vi "Prepare Acquisition.vi"(8 "error in (no error)":errorcluster, 10 "Flash Settings":T1={"Exposure Time (ms)"=100.0, "Binning"=enum."2x2", "Scan Mode"=0, "Frames to Acquire"=1000.0, "Pixel Correction"=FALSE, "Frames to Skip"=0, "File Path"=path "", "Duty cycle"=0.0, "ALEX"=FALSE, "Shutter Enable"=[], "fluidics trigger frame"=0, "Bit Depth"=0, "Image Width (px)"=0, "Image Height (px)"=0, "Horizontal Offset (px)"=0, "Vertical Offset (px)"=0} {"fluidics trigger frame" max=60000 step=1; "Exposure Time (ms)" min=1.0 max=10000.0 step=1.0}, 11 "Orca-Flash 4.0 in":refnum<class "Hamamatsu Camera.lvclass">) -> (0 "error out":errorcluster, 3 "Orca-Flash 4.0 out":refnum<class "Hamamatsu Camera.lvclass">)   [LabVIEW 2023, in "Hamamatsu Camera.lvlib" / "Hamamatsu Camera.lvclass"]
uses:
  Hamamatsu Camera.lvclass
  Resources/Type Defs/Camera Settings.ctl
  Hamamatsu Camera.lvclass/Hamamatsu Camera.ctl
  Resources/GLOBAL/GLOBAL Experiment Metadata.vi
  Resources/GLOBAL/GLOBAL Debug.vi
  Resources/GLOBAL/GLOBAL Time-critical.vi
  Hamamatsu Camera.lvlib
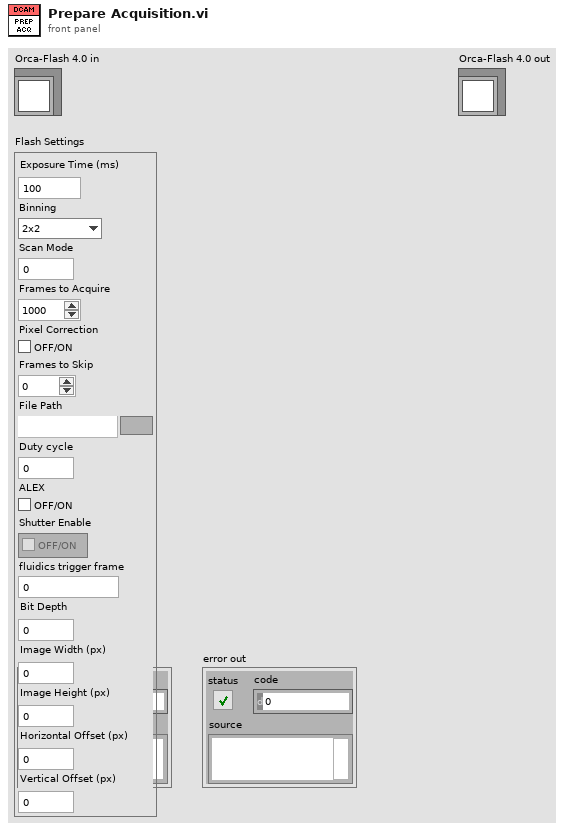
[diagram p1: front panel]
types:
  T1 = typedef "Camera Settings.ctl" = cluster{"Exposure Time (ms)":dbl, "Binning":enum16{"1x1", "2x2", "4x4"}, "Scan Mode":i32, "Frames to Acquire":dbl, "Pixel Correction":bool, "Frames to Skip":u32, "File Path":path, "Duty cycle":dbl, "ALEX":bool, "Shutter Enable":bool[], "fluidics trigger frame":u16, "Bit Depth":u16, "Image Width (px)":u16, "Image Height (px)":u16, "Horizontal Offset (px)":u16, "Vertical Offset (px)":u16}
  T2 = cluster{"Horizontal Offset":i32, "Vertical Offset":i32, "Horizontal Size":i32, "Vertical Size":i32}
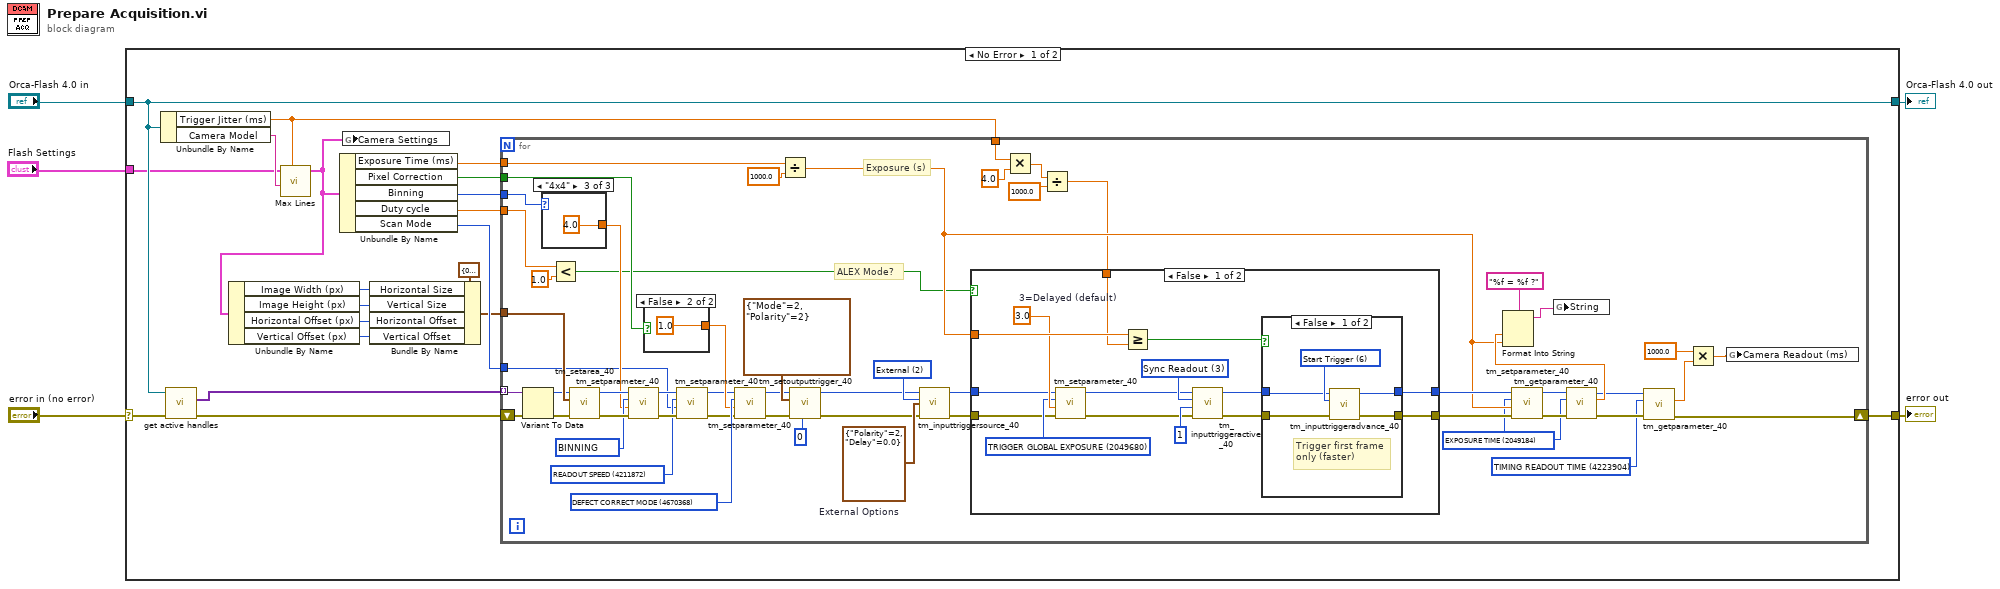
[diagram p0: block diagram]
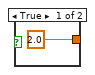
[diagram p2: hidden frame]
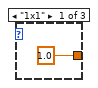
[diagram p3: hidden frame]
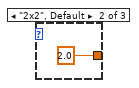
[diagram p4: hidden frame]
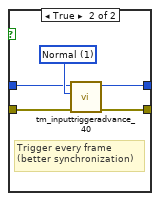
[diagram p5: hidden frame]
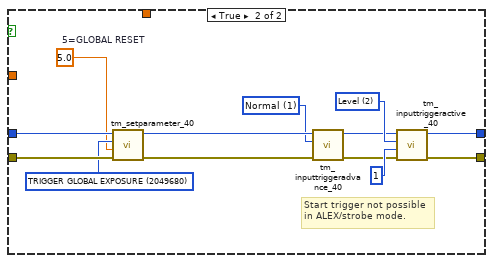
[diagram p6: hidden frame]
diagram:
  n1 = case shown="No Error" "error in (no error)" {
    selector: "error in (no error)" -> [w20 w125]
    tunnel: [w25 w125] -> w3
    tunnel: "Flash Settings" -> [w14 _]
    tunnel: "Orca-Flash 4.0 in" -> [w16 w124]
    tunnel: [w16 w124] -> w1
    frame No Error {
      n2 = Unbundle By Name(w16) -> ("Trigger Jitter (ms)"=w6:dbl, "Camera Model"=w15:string)
      n3 = call-dynamic "get active handles.vi"("error in (no error)"=w20, "Camera in"=w16) -> ("error out"=w21:errorcluster, "Handles"=w22:variant[])  [unwired: 5 in, 3 out]
      n4 = call "Max Lines.vi"("Trigger Jitter (ms)"=w6, "Camera Model"=w15, "Camera Setings In"=w14) -> ("Camera Settings Out"=w11:T1)  [unwired: 7 in, 1 out]
      n5 = Unbundle By Name(w11) -> ("Image Width (px)"=w10:u16, "Image Height (px)"=w9:u16, "Horizontal Offset (px)"=w8:u16, "Vertical Offset (px)"=w7:u16)
      n6 = Unbundle By Name(w11) -> ("Exposure Time (ms)"=w17:dbl, "Pixel Correction"=w24:bool, "Binning"=w23:enum16{"1x1", "2x2", "4x4"}, "Duty cycle"=w18:dbl, "Scan Mode"=w13:i32)
      n7 = global write "GLOBAL Experiment Metadata.vi" "Camera Settings"(w11) -> ()
      n8 = Bundle By Name(cluster=T2 {"Horizontal Offset"=0, "Vertical Offset"=0, "Horizontal Size"=0, "Vertical Size"=0} ("Sub Region"), "Horizontal Size"=w10, "Vertical Size"=w9, "Horizontal Offset"=w8, "Vertical Offset"=w7) -> (w12:T2)
      n9 = for {
        shift-right: [w34] -> w25
        shift-left: w21 -> [w41]
        tunnel: w22 -> [w39] mode=indexing
        tunnel: w17 -> [w49]
        tunnel: w24 -> [w48]
        tunnel: w23 -> [w47]
        tunnel: w18 -> [w46]
        tunnel: w12 -> [w43]
        tunnel: w13 -> [w42]
        tunnel: w6 -> [w28]
        w35 = u32 4223904 items=["SENSOR MODE"=4212128, "SENSOR MODE LINE BUNDLE HEIGHT"=4212192, "READOUT DIRECTION"=4211904, "BIT PER CHANNEL"=4342976, "EXPOSURE TIME"=2049184, "CONTRAST GAIN"=3163312, "BINNING"=4215968, "TIMING READOUT TIME"=4223904, "INTERNAL FRAME RATE"=4225952, "INTERNAL FRAME INTERVAL"=4225968, "INTERNAL LINE SPEED"=4226000, "IMAGE WIDTH"=4343200, "IMAGE HEIGHT"=4343216, "IMAGE ROWBYTES"=4343232, "IMAGE FRAMEBYTES"=4343248, "IMAGE PIXEL TYPE"=4343296] ("Parameter")
        w44 = u32 2049184 items=["SENSOR MODE"=4212128, "READOUT SPEED"=4211872, "READOUT DIRECTION"=4211904, "BIT PER CHANNEL"=4342976, "TRIGGER GLOBAL EXPOSURE"=2049680, "TRIGGER DELAY"=1066480, "SYNC READOUT SYSTEM BLANK"=1066528, "SENSOR COOLER STATUS"=2115280, "EXPOSURE TIME"=2049184, "DEFECT CORRECT MODE"=4670368, "BINNING"=4215968, "TIMING READOUT TIME"=4223904, "INTERNAL FRAME RATE"=4225952, "INTERNAL FRAME INTERVAL"=4225968, "INTERNAL LINE SPEED"=4226000, "INTERNAL LINE INTERVAL"=4226016, "IMAGE WIDTH"=4343200, "IMAGE HEIGHT"=4343216, "IMAGE ROWBYTES"=4343232, "IMAGE FRAMEBYTES"=4343248, "IMAGE PIXEL TYPE"=4343296, "NUMBER OF OUTPUT TRIGGER CONNECTOR"=1852320, "OUTPUT TRIGGER SOURCE[0]"=1852576, "OUTPUT TRIGGER SOURCE[1]"=1852832, "OUTPUT TRIGGER SOURCE[2]"=1853088, "OUTPUT TRIGGER POLARITY[0]"=1852592, "OUTPUT TRIGGER POLARITY[1]"=1852848, "OUTPUT TRIGGER POLARITY[2]"=1853104, "OUTPUT TRIGGER ACTIVE[0]"=1852608, "OUTPUT TRIGGER ACTIVE[1]"=1852864, "OUTPUT TRIGGER ACTIVE[2]"=1853120, "OUTPUT TRIGGER DELAY[0]"=1852624, "OUTPUT TRIGGER DELAY[1]"=1852880, "OUTPUT TRIGGER DELAY[2]"=1853136, "OUTPUT TRIGGER PERIOD[0]"=1852640, "OUTPUT TRIGGER PERIOD[1]"=1852896, "OUTPUT TRIGGER PERIOD[2]"=1853152, "OUTPUT TRIGGER KIND[0]"=1852656, "OUTPUT TRIGGER KIND[1]"=1852912, "OUTPUT TRIGGER KIND[2]"=1853168, "OUTPUT TRIGGER PRE HSYNC COUNT"=1852704] ("Parameter")
        w68 = 2 items=["Internal"=1, "External"=2, "Software"=3, "Master Pulse"=4] ("Source")
        w69 = cluster{"Polarity":i32, "Delay":dbl} {"Polarity"=2, "Delay"=0.0}  # External Options
        w72 = u32 4670368 items=["SENSOR MODE"=4212128, "READOUT SPEED"=4211872, "READOUT DIRECTION"=4211904, "BIT PER CHANNEL"=4342976, "TRIGGER GLOBAL EXPOSURE"=2049680, "TRIGGER DELAY"=1066480, "SYNC READOUT SYSTEM BLANK"=1066528, "SENSOR COOLER STATUS"=2115280, "EXPOSURE TIME"=2049184, "DEFECT CORRECT MODE"=4670368, "BINNING"=4215968, "TIMING READOUT TIME"=4223904, "INTERNAL FRAME RATE"=4225952, "INTERNAL FRAME INTERVAL"=4225968, "INTERNAL LINE SPEED"=4226000, "INTERNAL LINE INTERVAL"=4226016, "IMAGE WIDTH"=4343200, "IMAGE HEIGHT"=4343216, "IMAGE ROWBYTES"=4343232, "IMAGE FRAMEBYTES"=4343248, "IMAGE PIXEL TYPE"=4343296, "NUMBER OF OUTPUT TRIGGER CONNECTOR"=1852320, "OUTPUT TRIGGER SOURCE[0]"=1852576, "OUTPUT TRIGGER SOURCE[1]"=1852832, "OUTPUT TRIGGER SOURCE[2]"=1853088, "OUTPUT TRIGGER POLARITY[0]"=1852592, "OUTPUT TRIGGER POLARITY[1]"=1852848, "OUTPUT TRIGGER POLARITY[2]"=1853104, "OUTPUT TRIGGER ACTIVE[0]"=1852608, "OUTPUT TRIGGER ACTIVE[1]"=1852864, "OUTPUT TRIGGER ACTIVE[2]"=1853120, "OUTPUT TRIGGER DELAY[0]"=1852624, "OUTPUT TRIGGER DELAY[1]"=1852880, "OUTPUT TRIGGER DELAY[2]"=1853136, "OUTPUT TRIGGER PERIOD[0]"=1852640, "OUTPUT TRIGGER PERIOD[1]"=1852896, "OUTPUT TRIGGER PERIOD[2]"=1853152, "OUTPUT TRIGGER KIND[0]"=1852656, "OUTPUT TRIGGER KIND[1]"=1852912, "OUTPUT TRIGGER KIND[2]"=1853168, "OUTPUT TRIGGER PRE HSYNC COUNT"=1852704] ("Parameter")
        w73 = u32 4211872 items=["SENSOR MODE"=4212128, "READOUT SPEED"=4211872, "READOUT DIRECTION"=4211904, "BIT PER CHANNEL"=4342976, "TRIGGER GLOBAL EXPOSURE"=2049680, "TRIGGER DELAY"=1066480, "SYNC READOUT SYSTEM BLANK"=1066528, "SENSOR COOLER STATUS"=2115280, "EXPOSURE TIME"=2049184, "DEFECT CORRECT MODE"=4670368, "BINNING"=4215968, "TIMING READOUT TIME"=4223904, "INTERNAL FRAME RATE"=4225952, "INTERNAL FRAME INTERVAL"=4225968, "INTERNAL LINE SPEED"=4226000, "INTERNAL LINE INTERVAL"=4226016, "IMAGE WIDTH"=4343200, "IMAGE HEIGHT"=4343216, "IMAGE ROWBYTES"=4343232, "IMAGE FRAMEBYTES"=4343248, "IMAGE PIXEL TYPE"=4343296, "NUMBER OF OUTPUT TRIGGER CONNECTOR"=1852320, "OUTPUT TRIGGER SOURCE[0]"=1852576, "OUTPUT TRIGGER SOURCE[1]"=1852832, "OUTPUT TRIGGER SOURCE[2]"=1853088, "OUTPUT TRIGGER POLARITY[0]"=1852592, "OUTPUT TRIGGER POLARITY[1]"=1852848, "OUTPUT TRIGGER POLARITY[2]"=1853104, "OUTPUT TRIGGER ACTIVE[0]"=1852608, "OUTPUT TRIGGER ACTIVE[1]"=1852864, "OUTPUT TRIGGER ACTIVE[2]"=1853120, "OUTPUT TRIGGER DELAY[0]"=1852624, "OUTPUT TRIGGER DELAY[1]"=1852880, "OUTPUT TRIGGER DELAY[2]"=1853136, "OUTPUT TRIGGER PERIOD[0]"=1852640, "OUTPUT TRIGGER PERIOD[1]"=1852896, "OUTPUT TRIGGER PERIOD[2]"=1853152, "OUTPUT TRIGGER KIND[0]"=1852656, "OUTPUT TRIGGER KIND[1]"=1852912, "OUTPUT TRIGGER KIND[2]"=1853168, "OUTPUT TRIGGER PRE HSYNC COUNT"=1852704] ("Parameter")
        w77 = u32 4215968 items=["SENSOR MODE"=4212128, "READOUT SPEED"=4211872, "READOUT DIRECTION"=4211904, "BIT PER CHANNEL"=4342976, "TRIGGER GLOBAL EXPOSURE"=2049680, "TRIGGER DELAY"=1066480, "SYNC READOUT SYSTEM BLANK"=1066528, "SENSOR COOLER STATUS"=2115280, "EXPOSURE TIME"=2049184, "DEFECT CORRECT MODE"=4670368, "BINNING"=4215968, "TIMING READOUT TIME"=4223904, "INTERNAL FRAME RATE"=4225952, "INTERNAL FRAME INTERVAL"=4225968, "INTERNAL LINE SPEED"=4226000, "INTERNAL LINE INTERVAL"=4226016, "IMAGE WIDTH"=4343200, "IMAGE HEIGHT"=4343216, "IMAGE ROWBYTES"=4343232, "IMAGE FRAMEBYTES"=4343248, "IMAGE PIXEL TYPE"=4343296, "NUMBER OF OUTPUT TRIGGER CONNECTOR"=1852320, "OUTPUT TRIGGER SOURCE[0]"=1852576, "OUTPUT TRIGGER SOURCE[1]"=1852832, "OUTPUT TRIGGER SOURCE[2]"=1853088, "OUTPUT TRIGGER POLARITY[0]"=1852592, "OUTPUT TRIGGER POLARITY[1]"=1852848, "OUTPUT TRIGGER POLARITY[2]"=1853104, "OUTPUT TRIGGER ACTIVE[0]"=1852608, "OUTPUT TRIGGER ACTIVE[1]"=1852864, "OUTPUT TRIGGER ACTIVE[2]"=1853120, "OUTPUT TRIGGER DELAY[0]"=1852624, "OUTPUT TRIGGER DELAY[1]"=1852880, "OUTPUT TRIGGER DELAY[2]"=1853136, "OUTPUT TRIGGER PERIOD[0]"=1852640, "OUTPUT TRIGGER PERIOD[1]"=1852896, "OUTPUT TRIGGER PERIOD[2]"=1853152, "OUTPUT TRIGGER KIND[0]"=1852656, "OUTPUT TRIGGER KIND[1]"=1852912, "OUTPUT TRIGGER KIND[2]"=1853168, "OUTPUT TRIGGER PRE HSYNC COUNT"=1852704] ("Parameter")
        # "Exposure (s)"
        # "ALEX Mode?"
        n10 = Variant To Data(error in=w41, Variant=w39) -> (data=w38:u32, error out=w40:errorcluster)  [unwired: 1 in]
        n11 = case shown="\"4x4\"" w47 {
          tunnel: [1.0 ("Value in") 2.0 ("Value in") 4.0 ("Value in")] -> w76
          frame "1x1" {
          }
          frame "2x2", Default {
          }
          frame "4x4" {
          }
        }
        n12 = Less?(x=w46, y=1.0) -> (x < y?=w45:bool)
        n13 = call <userlib>:"tm_setarea_40.vi"("error in (no error)"=w40, "Sub Region"=w43, "Handle in"=w38) -> ("error out"=w79:errorcluster, "Handle out"=w78:u32)  [unwired: 7 in]
        n14 = call <userlib>:"tm_setparameter_40.vi"("error in (no error)"=w79, "Value in"=w76, "Parameter"=w77, "Handle in"=w78) -> ("error out"=w74:errorcluster, "Handle out"=w75:u32)  [unwired: 6 in]
        n15 = case shown="False" w48 {
          tunnel: [sgl 2.0 ("1 = OFF\n2 = ON") sgl 1.0 ("1 = OFF\n2 = ON")] -> w71
          frame True {
          }
          frame False {
          }
        }
        n16 = call <userlib>:"tm_setparameter_40.vi"("error in (no error)"=w74, "Value in"=w42, "Parameter"=w73, "Handle in"=w75) -> ("error out"=w55:errorcluster, "Handle out"=w56:u32)  [unwired: 6 in]
        n17 = call <userlib>:"tm_setparameter_40.vi"("error in (no error)"=w55, "Value in"=w71, "Parameter"=w72, "Handle in"=w56) -> ("error out"=w62:errorcluster, "Handle out"=w63:u32)  [unwired: 6 in]
        n18 = Divide(x=w49, y=1000.0) -> (x/y=w50:dbl)
        n19 = call <userlib>:"tm_setoutputtrigger_40.vi"("Port"=0, "error in (no error)"=w62, "Type"=cluster{"Mode":u32, "Polarity":u32} {"Mode"=2, "Polarity"=2}, "Handle in"=w63) -> ("error out"=w60:errorcluster, "Handle out"=w61:u32)  [unwired: 6 in]
        n20 = call <userlib>:"tm_inputtriggersource_40.vi"("error in (no error)"=w60, "External Options"=w69, "Source"=w68, "Handle in"=w61) -> ("error out"=w66:errorcluster, "Handle out"=w67:u32)  [unwired: 6 in]
        n21 = Multiply(x=w28, y=4.0) -> (x*y=w26:dbl)
        n22 = Divide(x=w26, y=1000.0) -> (x/y=w29:dbl)
        n23 = case shown="False" w45 {
          tunnel: [w99 w123] -> w54
          tunnel: [w98 w122] -> w53
          tunnel: w50 -> [w97 _]
          tunnel: w67 -> [w94 w121]
          tunnel: w66 -> [w93 w120]
          tunnel: w29 -> [w86 _]
          frame False {
            w91 = 3 items=["Edge"=1, "Level"=2, "Sync Readout"=3, "Point"=4] ("Active")
            w96 = 3.0  # 3=Delayed (default)
            w95 = u32 2049680 items=["SENSOR MODE"=4212128, "READOUT SPEED"=4211872, "READOUT DIRECTION"=4211904, "BIT PER CHANNEL"=4342976, "TRIGGER GLOBAL EXPOSURE"=2049680, "TRIGGER DELAY"=1066480, "SYNC READOUT SYSTEM BLANK"=1066528, "SENSOR COOLER STATUS"=2115280, "EXPOSURE TIME"=2049184, "DEFECT CORRECT MODE"=4670368, "BINNING"=4215968, "TIMING READOUT TIME"=4223904, "INTERNAL FRAME RATE"=4225952, "INTERNAL FRAME INTERVAL"=4225968, "INTERNAL LINE SPEED"=4226000, "INTERNAL LINE INTERVAL"=4226016, "IMAGE WIDTH"=4343200, "IMAGE HEIGHT"=4343216, "IMAGE ROWBYTES"=4343232, "IMAGE FRAMEBYTES"=4343248, "IMAGE PIXEL TYPE"=4343296, "NUMBER OF OUTPUT TRIGGER CONNECTOR"=1852320, "OUTPUT TRIGGER SOURCE[0]"=1852576, "OUTPUT TRIGGER SOURCE[1]"=1852832, "OUTPUT TRIGGER SOURCE[2]"=1853088, "OUTPUT TRIGGER POLARITY[0]"=1852592, "OUTPUT TRIGGER POLARITY[1]"=1852848, "OUTPUT TRIGGER POLARITY[2]"=1853104, "OUTPUT TRIGGER ACTIVE[0]"=1852608, "OUTPUT TRIGGER ACTIVE[1]"=1852864, "OUTPUT TRIGGER ACTIVE[2]"=1853120, "OUTPUT TRIGGER DELAY[0]"=1852624, "OUTPUT TRIGGER DELAY[1]"=1852880, "OUTPUT TRIGGER DELAY[2]"=1853136, "OUTPUT TRIGGER PERIOD[0]"=1852640, "OUTPUT TRIGGER PERIOD[1]"=1852896, "OUTPUT TRIGGER PERIOD[2]"=1853152, "OUTPUT TRIGGER KIND[0]"=1852656, "OUTPUT TRIGGER KIND[1]"=1852912, "OUTPUT TRIGGER KIND[2]"=1853168, "OUTPUT TRIGGER PRE HSYNC COUNT"=1852704] ("Parameter")
            n24 = call <userlib>:"tm_setparameter_40.vi"("error in (no error)"=w93, "Value in"=w96, "Parameter"=w95, "Handle in"=w94) -> ("error out"=w89:errorcluster, "Handle out"=w90:u32)  [unwired: 6 in]
            n25 = Greater Or Equal?(x=w97, y=w86) -> (x >= y?=w100:bool)
            n26 = call <userlib>:"tm_inputtriggeractive_40.vi"("error in (no error)"=w89, "Times"=1, "Active"=w91, "Handle in"=w90) -> ("error out"=w87:errorcluster, "Handle out"=w88:u32)  [unwired: 6 in]
            n27 = case shown="False" w100 {
              tunnel: [w105 w110] -> w99
              tunnel: [w104 w109] -> w98
              tunnel: w87 -> [w101 w106]
              tunnel: w88 -> [w102 w107]
              frame False {
                w103 = 6 items=["Normal"=1, "PIV"=3, "Start Trigger"=6, "Multigate"=7, "Multiframe"=8] ("option")
                # "Trigger first frame\nonly (faster)"
                n28 = call <userlib>:"tm_inputtriggeradvance_40.vi"("error in (no error)"=w101, "option"=w103, "Handle in"=w102) -> ("error out"=w104:errorcluster, "Handle out"=w105:u32)  [unwired: 7 in]
              }
              frame True {
                w108 = 1 items=["Normal"=1, "PIV"=3, "Start Trigger"=6, "Multigate"=7, "Multiframe"=8] ("option")
                # "Trigger every frame\n(better synchronization)"
                n29 = call <userlib>:"tm_inputtriggeradvance_40.vi"("error in (no error)"=w106, "option"=w108, "Handle in"=w107) -> ("error out"=w109:errorcluster, "Handle out"=w110:u32)  [unwired: 7 in]
              }
            }
          }
          frame True {
            w113 = 1 items=["Normal"=1, "PIV"=3, "Start Trigger"=6, "Multigate"=7, "Multiframe"=8] ("option")
            w114 = 2 items=["Edge"=1, "Level"=2, "Sync Readout"=3, "Point"=4] ("Active")
            w116 = 5.0  # 5=GLOBAL RESET
            w119 = u32 2049680 items=["SENSOR MODE"=4212128, "READOUT SPEED"=4211872, "READOUT DIRECTION"=4211904, "BIT PER CHANNEL"=4342976, "TRIGGER GLOBAL EXPOSURE"=2049680, "TRIGGER DELAY"=1066480, "SYNC READOUT SYSTEM BLANK"=1066528, "SENSOR COOLER STATUS"=2115280, "EXPOSURE TIME"=2049184, "DEFECT CORRECT MODE"=4670368, "BINNING"=4215968, "TIMING READOUT TIME"=4223904, "INTERNAL FRAME RATE"=4225952, "INTERNAL FRAME INTERVAL"=4225968, "INTERNAL LINE SPEED"=4226000, "INTERNAL LINE INTERVAL"=4226016, "IMAGE WIDTH"=4343200, "IMAGE HEIGHT"=4343216, "IMAGE ROWBYTES"=4343232, "IMAGE FRAMEBYTES"=4343248, "IMAGE PIXEL TYPE"=4343296, "NUMBER OF OUTPUT TRIGGER CONNECTOR"=1852320, "OUTPUT TRIGGER SOURCE[0]"=1852576, "OUTPUT TRIGGER SOURCE[1]"=1852832, "OUTPUT TRIGGER SOURCE[2]"=1853088, "OUTPUT TRIGGER POLARITY[0]"=1852592, "OUTPUT TRIGGER POLARITY[1]"=1852848, "OUTPUT TRIGGER POLARITY[2]"=1853104, "OUTPUT TRIGGER ACTIVE[0]"=1852608, "OUTPUT TRIGGER ACTIVE[1]"=1852864, "OUTPUT TRIGGER ACTIVE[2]"=1853120, "OUTPUT TRIGGER DELAY[0]"=1852624, "OUTPUT TRIGGER DELAY[1]"=1852880, "OUTPUT TRIGGER DELAY[2]"=1853136, "OUTPUT TRIGGER PERIOD[0]"=1852640, "OUTPUT TRIGGER PERIOD[1]"=1852896, "OUTPUT TRIGGER PERIOD[2]"=1853152, "OUTPUT TRIGGER KIND[0]"=1852656, "OUTPUT TRIGGER KIND[1]"=1852912, "OUTPUT TRIGGER KIND[2]"=1853168, "OUTPUT TRIGGER PRE HSYNC COUNT"=1852704] ("Parameter")
            # "Start trigger not possible\nin ALEX/strobe mode."
            n30 = call <userlib>:"tm_setparameter_40.vi"("error in (no error)"=w120, "Value in"=w116, "Parameter"=w119, "Handle in"=w121) -> ("error out"=w117:errorcluster, "Handle out"=w118:u32)  [unwired: 6 in]
            n31 = call <userlib>:"tm_inputtriggeradvance_40.vi"("error in (no error)"=w117, "option"=w113, "Handle in"=w118) -> ("error out"=w111:errorcluster, "Handle out"=w112:u32)  [unwired: 7 in]
            n32 = call <userlib>:"tm_inputtriggeractive_40.vi"("error in (no error)"=w111, "Times"=1, "Active"=w114, "Handle in"=w112) -> ("error out"=w122:errorcluster, "Handle out"=w123:u32)  [unwired: 6 in]
          }
        }
        n33 = call <userlib>:"tm_setparameter_40.vi"("error in (no error)"=w53, "Value in"=w50, "Parameter"=w44, "Handle in"=w54) -> ("error out"=w52:errorcluster, "Handle out"=w51:u32)  [unwired: 6 in]
        n34 = call <userlib>:"tm_getparameter_40.vi"("error in (no error)"=w52, "Parameter"=w44, "Handle in"=w51) -> ("error out"=w37:errorcluster, "Value out"=w57:dbl, "Handle out"=w36:u32)  [unwired: 6 in]
        n35 = Format Into String(format string="%f = %f ?", w57, w50) -> (resulting string=w59:string)  [unwired: 2 in, 1 out]
        n36 = global write "GLOBAL Debug.vi" "String"(w59) -> ()
        n37 = call <userlib>:"tm_getparameter_40.vi"("error in (no error)"=w37, "Parameter"=w35, "Handle in"=w36) -> ("error out"=w34:errorcluster, "Value out"=w32:dbl)  [unwired: 6 in, 1 out]
        n38 = Multiply(x=1000.0, y=w32) -> (x*y=w33:dbl)
        n39 = global write "GLOBAL Time-critical.vi" "Camera Readout (ms)"(w33) -> ()
      }
    }
    frame Error {
    }
  }
  "error out" <- w3
  "Orca-Flash 4.0 out" <- w1
